vi "Generate Circular Arc Points.vi"(6 "Index":i32, 9 "Circle Info":T2, 11 "Speeds":T1={"maxV (fps)"=20.0, "Accel Limit (fps^2)"=20.0, "Initial V (fps)"=0.0, "Sample Period (s)"=0.02, "Accel Dist (ft)"=0.0, "Decel Dist (ft)"=0.0}) -> (1 "Final Position":cluster{dbl, dbl, dbl}, 2 "Trajectory Segment":T3, 3 "Speeds Out":T1={"maxV (fps)"=0.0, "Accel Limit (fps^2)"=0.0, "Initial V (fps)"=0.0, "Sample Period (s)"=0.02, "Accel Dist (ft)"=0.0, "Decel Dist (ft)"=0.0})   [LabVIEW 2023]
panel:
  out "Point Arrays":cluster{dbl[], dbl[], dbl[]}
  out "XY Graph":cluster{dbl, dbl}[](graph)
  out "Segment Time (s)":dbl
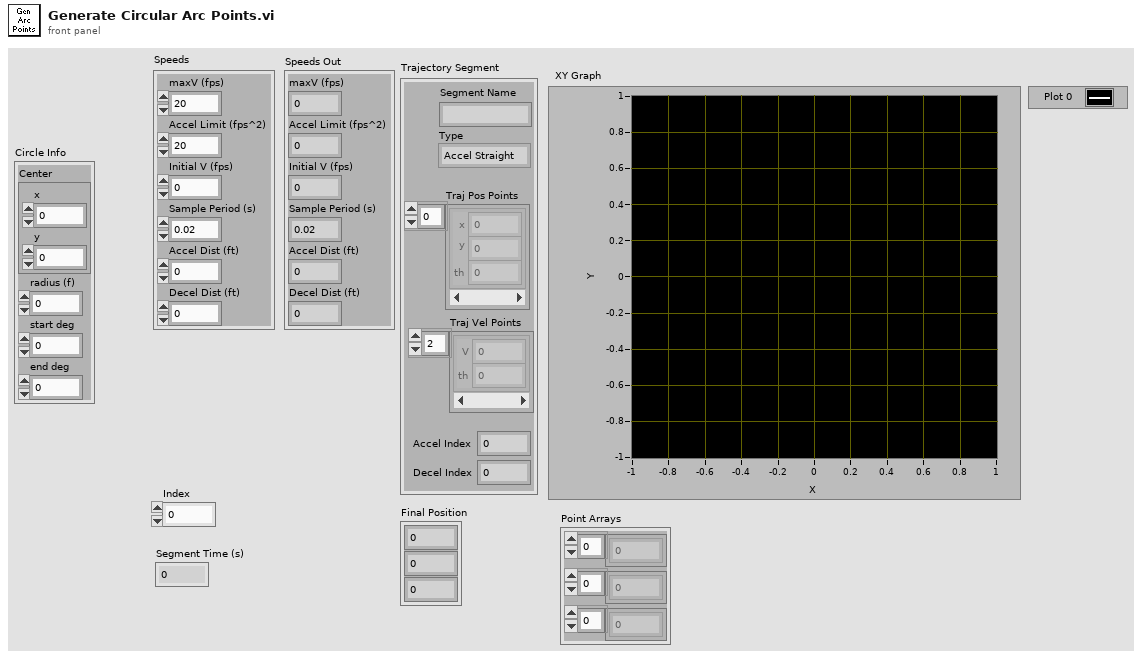
[diagram p1: front panel]
types:
  T1 = cluster{"maxV (fps)":dbl, "Accel Limit (fps^2)":dbl, "Initial V (fps)":dbl, "Sample Period (s)":dbl, "Accel Dist (ft)":dbl, "Decel Dist (ft)":dbl}
  T2 = cluster{"Center":cluster{"x":dbl, "y":dbl}, "radius (f)":dbl, "start deg":dbl, "end deg":dbl}
  T3 = cluster{"Segment Name":string, "Type":enum16{"Accel Straight", "Const Straight", "Blend", "Circle"}, "Traj Pos Points":cluster{"x":dbl, "y":dbl, "th":dbl}[], "Traj Vel Points":cluster{"V":dbl, "th":dbl}[], "Accel Index":i32, "Decel Index":i32}
  T4 = enum16{"Accel Straight", "Const Straight", "Blend", "Circle"}
  T5 = cluster{string, "Type":enum16{"Accel Straight", "Const Straight", "Blend", "Circle"}, cluster{dbl, dbl, dbl}[], cluster{"maxV (fps)":dbl, dbl}[], "Accel Index":i32, "Decel Index":i32}
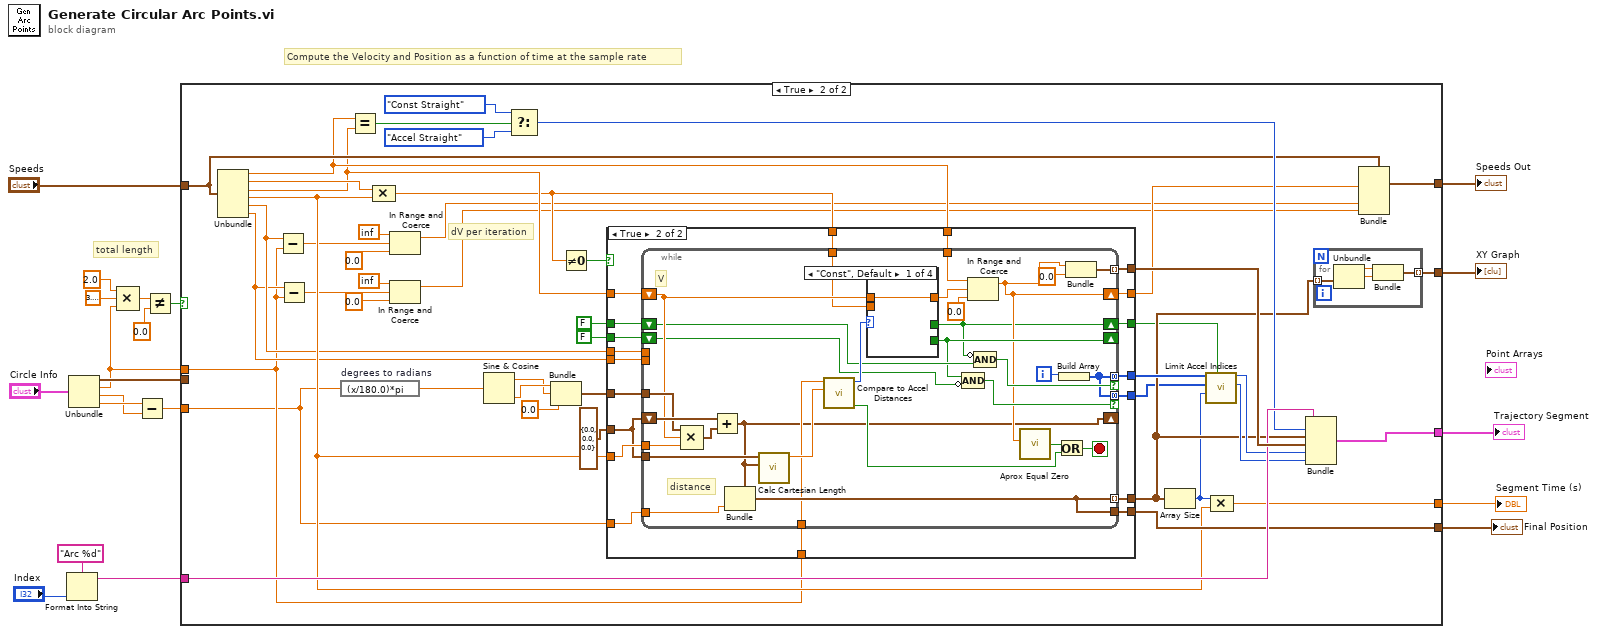
[diagram p0: block diagram]
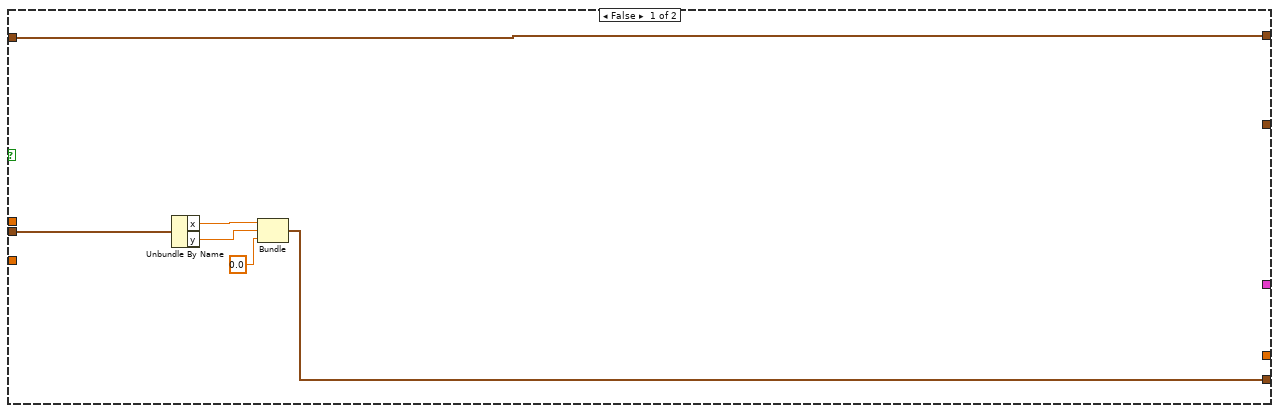
[diagram p2: hidden frame]
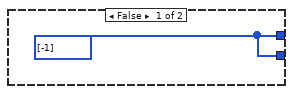
[diagram p3: hidden frame]
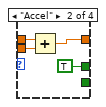
[diagram p4: hidden frame]
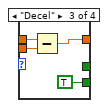
[diagram p5: hidden frame]
diagram:
  # "total length"
  # "Compute the Velocity and Position as a function of time at the sample rate"
  n1 = Format Into String(format string="Arc %d", "Index") -> (resulting string=w11:string)  [unwired: 2 in, 1 out]
  n2 = Unbundle("Circle Info") -> ("Center"=w13:cluster{"x":dbl, "y":dbl}, "radius (f)"=w7:dbl, "start deg"=w5:dbl, "end deg"=w6:dbl)
  n3 = Compound Arithmetic op=MULTIPLY(2.0 ("value"), 3.141592653589793, w7) -> (w4:dbl)
  n4 = Subtract(x=w6, y=w5) -> (x-y=w1:dbl)
  n5 = Not Equal?(x=w4, y=0.0) -> (x != y?=w2:bool)
  n6 = case shown="True" w2 {
    tunnel: [_ w72] -> w20
    tunnel: w11 -> [_ w66]
    tunnel: [_ w62] -> w19
    tunnel: [w21 w61] -> w18
    tunnel: [_ w59] -> w17
    tunnel: "Speeds" -> [w26 w57]
    tunnel: [w26 w55] -> w15
    tunnel: w13 -> [w25 _]
    tunnel: w7 -> [_ w30]
    tunnel: w1 -> [_ w27]
    frame False {
      n7 = Unbundle By Name(w25) -> ("x"=w24:dbl, "y"=w23:dbl)
      n8 = Bundle("x"=w24, "y"=w23, 0.0) -> (w21:cluster{"x":dbl, "y":dbl, dbl})  [unwired: 1 in]
    }
    frame True {
      # "dV per iteration"
      n9 = Unbundle(w57) -> ("maxV (fps)"=w54:dbl, "Accel Limit (fps^2)"=w58:dbl, "Initial V (fps)"=w53:dbl, "Sample Period (s)"=w51:dbl, "Accel Dist (ft)"=w41:dbl, "Decel Dist (ft)"=w36:dbl)
      n10 = Subtract(x=w41, y=w30) -> (x-y=w45:dbl)
      n11 = Subtract(x=w36, y=w30) -> (x-y=w37:dbl)
      n12 = expression code="(x/180.0)*pi" "degrees to radians"(w27) -> (w60:dbl)
      n13 = Equal?(x=w54, y=w53) -> (x = y?=w52:bool)
      n14 = Compound Arithmetic op=MULTIPLY(w58, w51) -> (w50:dbl)
      n15 = In Range and Coerce(upper limit=inf, x=w45, lower limit=0.0) -> (coerced(x)=w44:dbl)  [unwired: 1 out]
      n16 = In Range and Coerce(upper limit=inf, x=w37, lower limit=0.0) -> (coerced(x)=w28:dbl)  [unwired: 1 out]
      n17 = Sine & Cosine(0:w60) -> (1:w67:dbl, 2:w68:dbl)
      n18 = Select(t=T4."Const Straight" ("Type"), s=w52, f=T4."Accel Straight" ("Type")) -> (s? t:f=w63:T4)
      n19 = Bundle(w68, w67, 0.0) -> (w70:cluster{dbl, dbl, dbl})  [unwired: 1 in]
      n20 = Not Equal To 0?(x=w50) -> (x != 0?=w49:bool)
      n21 = case shown="True" w49 {
        tunnel: [_ w96] -> w71
        tunnel: w70 -> [_ w95]
        tunnel: [_ w94] -> w61
        tunnel: w27 -> [_ w93]
        tunnel: [_ w92] -> w34
        tunnel: [_ w91] -> w56
        tunnel: w54 -> [_ w90]
        tunnel: w53 -> [_ w89]
        tunnel: w50 -> [_ w88]
        tunnel: w51 -> [_ w87]
        tunnel: cluster{"x":dbl, "y":dbl, dbl} {"x"=0.0, "y"=0.0, 0.0} ("Center") -> [_ w86]
        tunnel: w30 -> [_ w85]
        tunnel: FALSE -> [_ w84]
        tunnel: [w77 w83] -> w42
        tunnel: w41 -> [_ w82]
        tunnel: w36 -> [_ w81]
        tunnel: FALSE -> [_ w80]
        tunnel: [w77 w79] -> w33
        tunnel: [_ w78] -> w31
        frame False {
          w77 = i32[] [-1]
        }
        frame True {
          n22 = while {
            tunnel: [w118] -> w92 mode=indexing
            tunnel: w88 -> [w110]
            shift-right: [w101] -> w91
            shift-left: w89 -> [w112]
            tunnel: [w124] -> w96 mode=indexing
            tunnel: w87 -> [w120]
            tunnel: w95 -> [w121]
            tunnel: w93 -> [w125]
            tunnel: [w118] -> w94
            tunnel: w90 -> [w123]
            tunnel: w85 -> [w114]
            shift-right: [w98] -> _
            shift-left: w86 -> [w122]
            tunnel: w86 -> [w119]
            shift-right: [w97] -> w78
            shift-left: w84 -> [w109]
            tunnel: [w105] -> w83 mode=concatenating if=w108
            tunnel: w82 -> [_]
            tunnel: w81 -> [_]
            shift-right: [w106] -> _
            shift-left: w80 -> [w107]
            tunnel: [w105] -> w79 mode=concatenating if=w104
            i -> [w117]
            stop <- w102 stop-if-true
            # "V"
            # "distance"
            n23 = Compound Arithmetic op=MULTIPLY(w121, w112, w120) -> (w99:cluster{dbl, dbl, dbl})
            n24 = Add(x=w122, y=w99) -> (x+y=w98:cluster{dbl, dbl, dbl})
            n25 = Bundle(cluster=w98, w125) -> (w118:cluster{dbl, dbl, dbl})  [unwired: 2 in]
            n26 = call "Calc Cartesian Length.vi"("Point 2"=w98, "Point 1"=w119) -> ("Length (f)"=w115:dbl)  [unwired: 8 in, 1 out]
            n27 = call "Compare to Accel Distances.vi"("Current  Length"=w115, "Total Segment Length"=w114) -> ("End Loop"=w103:bool, "Action"=w113:enum16{"Const", "Accel", "Decel", "Both"})  [unwired: 6 in, 2 out]
            n28 = case shown="\"Const\", Default" w113 {
              tunnel: w112 -> [w127 w131 w135 w136]
              tunnel: [w127 w129 w133 w136] -> w111
              tunnel: w110 -> [_ w130 w134 _]
              tunnel: [_ TRUE _ _] -> w97
              tunnel: [_ _ TRUE _] -> w106
              frame "Const", Default {
              }
              frame "Accel" {
                n29 = Add(x=w131, y=w130) -> (x+y=w129:dbl)
              }
              frame "Decel" {
                n30 = Subtract(x=w135, y=w134) -> (x-y=w133:dbl)
              }
              frame "Both" {
              }
            }
            n31 = Compound Arithmetic op=AND(w106, invert w107) -> (w104:bool)
            n32 = In Range and Coerce(upper limit=w123, x=w111, lower limit=0.0) -> (coerced(x)=w101:dbl)  [unwired: 1 out]
            n33 = Compound Arithmetic op=AND(invert w97, w109) -> (w108:bool)
            n34 = call "Aprox Equal Zero.vi"("x"=w101) -> ("Boolean"=w100:bool)  [unwired: 10 in]
            n35 = Or(x=w100, y=w103) -> (x .or. y?=w102:bool)
            n36 = Build Array(w117) -> (w105:i32[])
            n37 = Bundle("maxV (fps)"=w101, 0.0) -> (w124:cluster{"maxV (fps)":dbl, dbl})  [unwired: 1 in]
          }
        }
      }
      n38 = Array Size(array=w34) -> (size(s)=w32:i32)
      n39 = call "Limit Accel Indices.vi"("Last Accel"=w31, "Size"=w32, "Decel"=w33, "Accel"=w42) -> ("Decel Index"=w40:i32, "Accel Index"=w43:i32)  [unwired: 6 in]
      n40 = Compound Arithmetic op=MULTIPLY(w32, w51) -> (w62:dbl)
      n41 = Bundle(w66, "Type"=w63, w34, w71, "Accel Index"=w43, "Decel Index"=w40) -> (w72:T5)  [unwired: 1 in]
      n42 = for {
        tunnel: w34 -> [w76] mode=indexing
        tunnel: [w73] -> w59 mode=indexing
        n43 = Unbundle(w76) -> (w75:dbl, w74:dbl)  [unwired: 1 out]
        n44 = Bundle(w75, w74) -> (w73:cluster{dbl, dbl})  [unwired: 1 in]
      }
      n45 = Bundle(cluster=w57, "Initial V (fps)"=w56, "Accel Dist (ft)"=w44, "Decel Dist (ft)"=w28) -> (w55:T1)  [unwired: 3 in]
    }
  }
  "Trajectory Segment" <- w20
  "Segment Time (s)" <- w19
  "Final Position" <- w18
  "XY Graph" <- w17
  "Speeds Out" <- w15
